vi "GetSystemTheme.vi"(8 "No Error":errorcluster) -> (0 "Error Out":errorcluster, 3 "SystemTheme":T1)   [LabVIEW 2026, in "SDL3.lvlib" / "Video.lvlib"]
doc: "<B>Summary</B>\nGet parent of a window."
uses:
  Video.lvlib
  SystemTheme--enum.ctl
  Lib/SDL3.dll
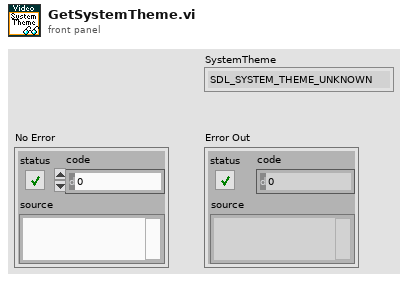
[diagram p1: front panel]
types:
  T1 = typedef "SDL3.lvlib/Video.lvlib/SystemTheme--enum.ctl" = enum32{"SDL_SYSTEM_THEME_UNKNOWN", "SDL_SYSTEM_THEME_LIGHT", "SDL_SYSTEM_THEME_DARK"}
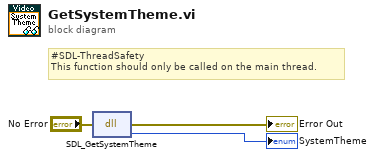
[diagram p0: block diagram]
diagram:
  # "#SDL-ThreadSafety\nThis function should only be called on the main thread."
  n1 = dll-call lib="C:/Users/saukko/Dev/LV-SDL3/Sources/SDL3/Lib/SDL3.*" fn="SDL_GetSystemTheme"(error in="No Error") -> (error out=→"Error Out":errorcluster, "return type"=→"SystemTheme":u32)  [unwired: 2 in, 1 out]
